vi "Check ID for Minor Frame.vi"(7 "ID":string, 8 "error in (no error)":errorcluster, 11 "Major Frame in":refnum<class "Major Frame.lvclass">) -> (0 "error out":errorcluster, 2 "Minor Frame Found?":bool, 3 "Major Frame out":refnum<class "Major Frame.lvclass">, 5 "Minor Frame":refnum<class "Minor Frame.lvclass">)   [LabVIEW 2020, in "BCI-1553 API.lvlib" / "Major Frame.lvclass"]
doc: "Verifies if an ID is a Minor Frame."
uses:
  Major Frame.lvclass
  Minor Frame/Minor Frame.lvclass
  Major Frame.lvclass/Major Frame.ctl
  Dependencies/Registry/Registry.lvclass/Registry.ctl
  Dependencies/Registry/Registry.lvclass
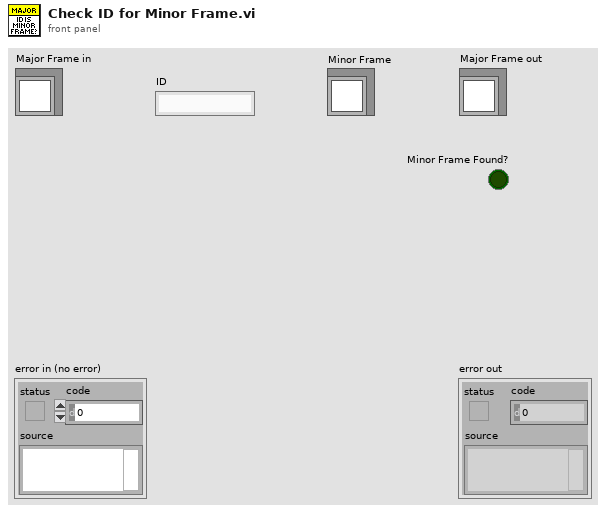
[diagram p1: front panel]
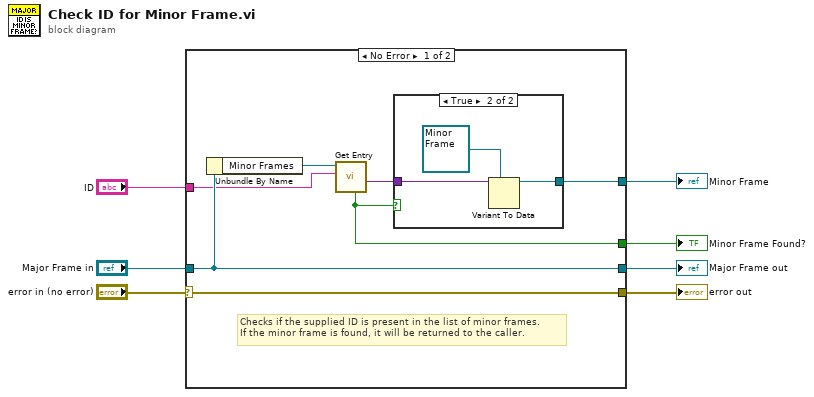
[diagram p0: block diagram]
diagram:
  n1 = case shown="No Error" "error in (no error)" {
    selector: "error in (no error)" -> [w14 w19]
    tunnel: [w14 w19] -> w1
    tunnel: [w13 w18] -> w2
    tunnel: "Major Frame in" -> [w13 w18]
    tunnel: "ID" -> [w11 _]
    tunnel: [w9 _] -> w3
    tunnel: [w8 _] -> w4
    frame No Error {
      # "Checks if the supplied ID is present in the list of minor frames.\nIf the minor frame is found, it will be returned to the caller."
      n2 = Unbundle By Name(w13) -> ("Minor Frames"=w12:refnum<class "Registry.lvclass">)
      n3 = call "Get Entry.vi"("Key"=w11, "Registry in"=w12) -> ("Value"=w10:variant, "Found?"=w9:bool)  [unwired: 6 in, 2 out]
      n4 = case shown="True" w9 {
        tunnel: w10 -> [_ w17]
        tunnel: [_ w16] -> w8
        frame False {
        }
        frame True {
          n5 = Variant To Data(type=refnum<class "Minor Frame.lvclass"> refnum ("Minor Frame"), Variant=w17) -> (data=w16:refnum<class "Minor Frame.lvclass">)  [unwired: 1 in, 1 out]
        }
      }
    }
    frame Error {
    }
  }
  "error out" <- w1
  "Major Frame out" <- w2
  "Minor Frame Found?" <- w3
  "Minor Frame" <- w4
